vi "svacg_Low-Level Limit Testing Time-WDT.vi"(6 "limit test config":T1={"pass region"=0, "include UL"=TRUE, "include LL"=TRUE} {"pass region" items=["inside limits", "outside limits"]}, 8 "error in":errorcluster, 9 "lower limit":waveform(dbl)={"t0"=timestamp(0 s since 1904-01-01), "dt"=0.0, "Y"=[]}, 10 "upper limit":waveform(dbl)={"t0"=timestamp(0 s since 1904-01-01), "dt"=0.0, "Y"=[]}, 11 "signal in":waveform(dbl)) -> (0 "error out":errorcluster, 1 "output values":waveform(dbl)[](array[waveform]), 2 "test results":bool[](array[boolean]), 3 "test passed?":bool, 4 "clearance":T2 {"min clearance" format="%.2p"; "clearance LL" format="%.2p"; "clearance UL" format="%.2p"}, 5 "failures":cluster{"x values":dbl[], "y values":dbl[]} {"y values" format="%.2p"; "x values" format="%.2p"})   [LabVIEW 2017]
uses:
  <vilib>/measure/NI_MABase.lvlib
  <vilib>/measure/NI_MAPro.lvlib
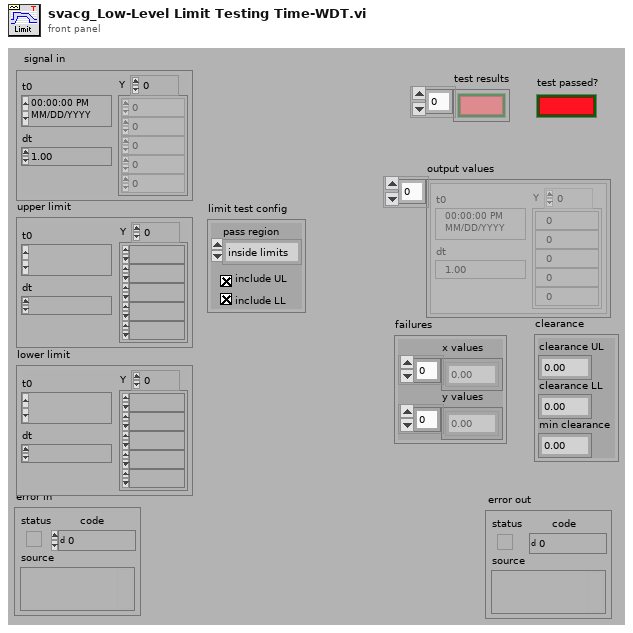
[diagram p1: front panel]
types:
  T1 = cluster{"pass region":i32, "include UL":bool, "include LL":bool}
  T2 = cluster{"clearance UL":dbl, "clearance LL":dbl, "min clearance":dbl}
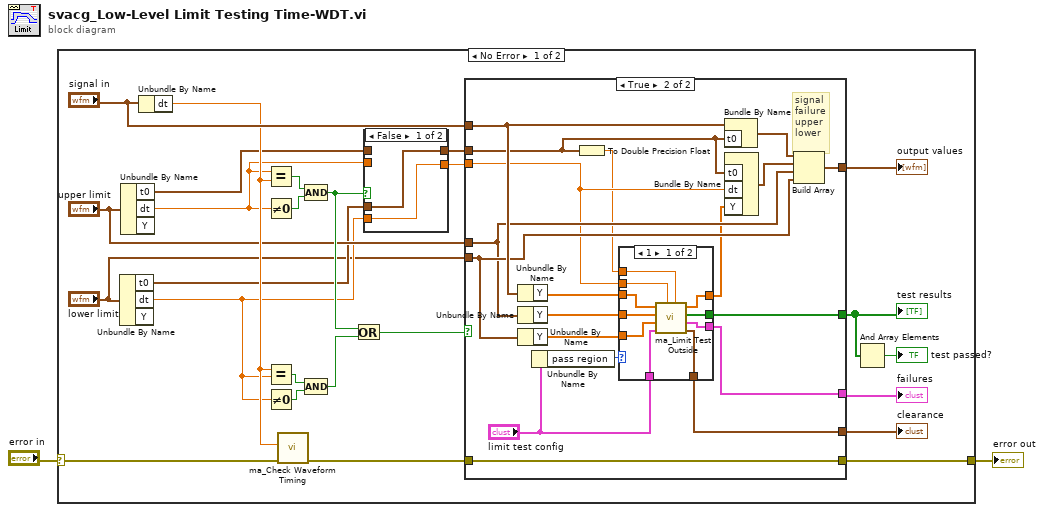
[diagram p0: block diagram]
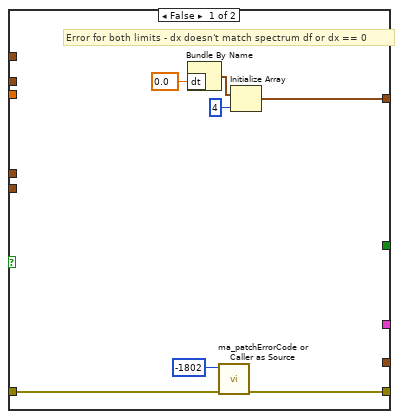
[diagram p3: hidden frame]
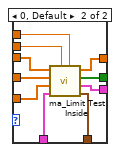
[diagram p4: hidden frame]
diagram:
  n1 = case shown="No Error" "error in" {
    selector: "error in" -> [w11 w78]
    tunnel: [w12 w78] -> w1
    frame No Error {
      n2 = Unbundle By Name("lower limit") -> ("t0"=w5:timestamp, "dt"=w4:dbl)  [unwired: 1 out]
      n3 = Unbundle By Name("upper limit") -> ("t0"=w7:timestamp, "dt"=w8:dbl)  [unwired: 1 out]
      n4 = Unbundle By Name("signal in") -> ("dt"=w10:dbl)
      n5 = Equal?(x=w8, y=w10) -> (x = y?=w26:bool)
      n6 = Not Equal To 0?(x=w8) -> (x != 0?=w25:bool)
      n7 = Equal?(x=w10, y=w4) -> (x = y?=w27:bool)
      n8 = Not Equal To 0?(x=w4) -> (x != 0?=w24:bool)
      n9 = call <vilib>:"ma_Check Waveform Timing.vi"("error in (no error)"=w11, "dt"=w10) -> ("error out"=w9:errorcluster)  [unwired: 8 in, 1 out]
      n10 = Compound Arithmetic op=AND(w26, w25) -> (w20:bool)
      n11 = Compound Arithmetic op=AND(w27, w24) -> (w21:bool)
      n12 = Or(x=w20, y=w21) -> (x .or. y?=w22:bool)
      n13 = case shown="False" w20 {
        tunnel: w7 -> [_ w31]
        tunnel: w8 -> [_ w30]
        tunnel: w5 -> [w29 _]
        tunnel: w4 -> [w28 _]
        tunnel: [w29 w31] -> w19
        tunnel: [w28 w30] -> w18
        frame False {
        }
        frame True {
        }
      }
      n14 = case shown="True" w22 {
        tunnel: [_ w57] -> w16
        tunnel: "upper limit" -> [_ w48]
        tunnel: "lower limit" -> [_ w49]
        tunnel: "signal in" -> [_ w51]
        tunnel: w19 -> [_ w39]
        tunnel: w18 -> [_ w45]
        tunnel: w9 -> [w36 w52]
        tunnel: [w35 w52] -> w12
        tunnel: [w34 w42] -> w17
        tunnel: [_ w56] -> w14
        tunnel: [_ w55] -> w13
        frame False {
          # "Error for both limits - dx doesn't match spectrum df or dx == 0"
          n15 = Bundle By Name("dt"=0.0) -> (w32:waveform(dbl))  [unwired: 1 in]
          n16 = call <vilib>:"ma_patchErrorCode or Caller as Source.vi"("error in (no error)"=w36, "error code"=-1802 ("Error Code")) -> ("error out"=w35:errorcluster)  [unwired: 9 in]
          n17 = Initialize Array(w32, 4 ("dimension size")) -> (w34:waveform(dbl)[])
        }
        frame True {
          # "signal\nfailure\nupper\nlower"
          n18 = Unbundle By Name(w51) -> ("Y"=w50:dbl[])
          n19 = Unbundle By Name(w48) -> ("Y"=w47:dbl[])
          n20 = Unbundle By Name(w49) -> ("Y"=w46:dbl[])
          n21 = Unbundle By Name("limit test config") -> ("pass region"=w53:i32)
          n22 = To Double Precision Float(number=w39) -> (double precision float=w40:dbl)
          n23 = case shown="1" w53 {
            tunnel: [w67 w71] -> w57
            tunnel: w47 -> [w66 w77]
            tunnel: w46 -> [w65 w76]
            tunnel: [w64 w75] -> w44
            tunnel: [w63 w74] -> w56
            tunnel: [w62 w73] -> w55
            tunnel: "limit test config" -> [w61 w72]
            tunnel: w40 -> [w60 w70]
            tunnel: w45 -> [w59 w69]
            tunnel: w50 -> [w58 w68]
            frame 1 {
              n24 = call <vilib>:"ma_Limit Test Outside.vi"("x0"=w60, "dx"=w59, "limit test config"=w61, "lower"=w65, "upper"=w66, "signal"=w58) -> ("clearance"=w62:T2, "failures"=w63:cluster{"x values":dbl[], "y values":dbl[]}, "test results"=w67:bool[], "Y"=w64:dbl[])  [unwired: 2 in]
            }
            frame 0, Default {
              n25 = call <vilib>:"ma_Limit Test Inside.vi"("x0"=w70, "dx"=w69, "limit test config"=w72, "lower"=w76, "upper"=w77, "signal"=w68) -> ("clearance"=w73:T2, "failures"=w74:cluster{"x values":dbl[], "y values":dbl[]}, "test results"=w71:bool[], "Y"=w75:dbl[])  [unwired: 2 in]
            }
          }
          n26 = Bundle By Name(cluster=w51, "t0"=w39) -> (w41:waveform(dbl))
          n27 = Bundle By Name("t0"=w39, "dt"=w45, "Y"=w44) -> (w43:waveform(dbl))  [unwired: 1 in]
          n28 = Build Array(w41, w43, w48, w49) -> (w42:waveform(dbl)[])
        }
      }
      "output values" <- w17
      "test results" <- w16
      "failures" <- w14
      "clearance" <- w13
      n29 = And Array Elements(Boolean array=w16) -> (logical AND=→"test passed?":bool)
    }
    frame Error {
    }
  }
  "error out" <- w1
